vi "Add Item.vi"(8 "error in (no error)":errorcluster, 10 "ItemInfo":T1={"Parent Tag (\"\")"="", "Child Position (-1=End)"=-1, "Left Cell String (\"\" = Same as Child Tag)"="", "Child Text[]"=[], "Child Tag"="", "Child Only? (F)"=FALSE}, 11 "Tree in":refnum<class "TreeSelection.lvclass">) -> (0 "error out":errorcluster, 2 "Add Item Tag":string, 3 "Tree out":refnum<class "TreeSelection.lvclass">)   [LabVIEW 2015, in "TreeSelection.lvclass"]
doc: "<b> </b> <b> </b>\n©2016 Q Software Innovations, LLC (QSI)\nwritten by Quentin Alldredge\nproduced in LabVIEW 2015\n\nsupport@qsoftwareinnovations.com\nwww.qsoftwareinnovations.com\n\nAll rights reserved.\n\nRedistribution and use in source and binary forms, with or without modification, are permitted provided that the following conditions are met:\n\n * Redistributions of source code must retain the above copyright notice, this list of conditions and the following disclaimer.\n * Redistributions in binary form must reproduce the above copyright notice, this list of conditions and the following disclaimer in the documentation and/or other materials provided with the distribution.\n * Neither the name of Q Software Innovations, LLC. nor the names of its contributors may be used to endorse or promote products derived from this software without specific prior written permission.\n\nTHIS SOFTWARE IS PROVIDED BY THE COPYRIGHT HOLDERS AND CONTRIBUTORS \"AS IS\" AND ANY EXPRESS OR IMPLIED WARRANTIES, INCLUDING, BUT NOT LIMITED TO, THE IMPLIED WARRANTIES OF MERCHANTABILITY AND FITNESS FOR A PARTICULAR PURPOSE ARE DISCLAIMED. IN NO EVENT SHALL THE COPYRIGHT OWNER OR CONTRIBUTORS BE LIABLE FOR ANY DIRECT, INDIRECT, INCIDENTAL, SPECIAL, EXEMPLARY, OR CONSEQUENTIAL DAMAGES (INCLUDING, BUT NOT LIMITED TO, PROCUREMENT OF SUBSTITUTE GOODS OR SERVICES; LOSS OF USE, DATA, OR PROFITS; OR BUSINESS INTERRUPTION) HOWEVER CAUSED AND ON ANY THEORY OF LIABILITY, WHETHER IN CONTRACT, STRICT LIABILITY, OR TORT (INCLUDING NEGLIGENCE OR OTHERWISE) ARISING IN ANY WAY OUT OF THE USE OF THIS SOFTWARE, EVEN IF ADVISED OF THE POSSIBILITY OF SUCH DAMAGE."
uses:
  TreeSelection.lvclass
  TreeControl/Add Item Info Cluster.ctl
  TreeControl/TreeControl.lvclass
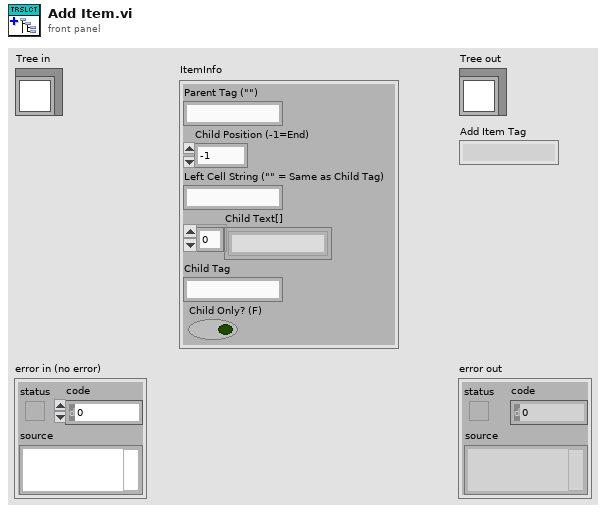
[diagram p1: front panel]
types:
  T1 = typedef "TreeControl.lvclass/Add Item Info Cluster.ctl" = cluster{"Parent Tag (\"\")":string, "Child Position (-1=End)":i32, "Left Cell String (\"\" = Same as Child Tag)":string, "Child Text[]":string[], "Child Tag":string, "Child Only? (F)":bool}
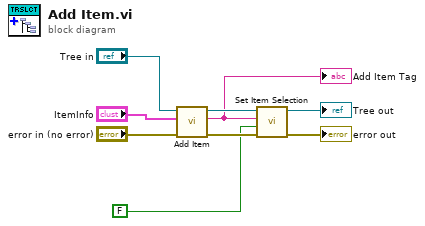
[diagram p0: block diagram]
diagram:
  n1 = call-parent "Add Item.vi"("error in (no error)"="error in (no error)", "ItemInfo"="ItemInfo", "Tree in"="Tree in") -> ("error out"=w3:errorcluster, "Add Item Tag"=w5:string, "Tree (dup)"=w7:refnum<class "TreeSelection.lvclass">)  [unwired: 6 in]
  "Add Item Tag" <- w5
  n2 = call-dynamic "Set Item Selection.vi"("error in (no error)"=w3, "Selected?"=FALSE, "Tag"=w5, "TreeSelection in"=w7) -> ("error out"=→"error out":errorcluster, "TreeSelection out"=→"Tree out":refnum<class "TreeSelection.lvclass">)  [unwired: 6 in]
